vi "dosimat876_initialize.vi"(2 "error in":errorcluster, 3 "Dosimat Port In":refnum<visa-resource-name>="COM1") -> (1 "Dosimat Out":T1={"Dosimat Port out"="COM1", "Error out"={"status"=FALSE, "code"=0, "source"=""}})   [LabVIEW 2010]
uses:
  <vilib>/Instr/_visa.llb/VISA Configure Serial Port (Instr).vi
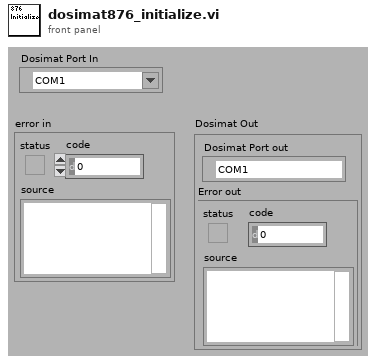
[diagram p1: front panel]
types:
  T1 = cluster{"Dosimat Port out":refnum<visa-resource-name>, "Error out":errorcluster}
  T2 = cluster{"Dosimat Port Out":refnum<visa-resource-name>, "error out":errorcluster}
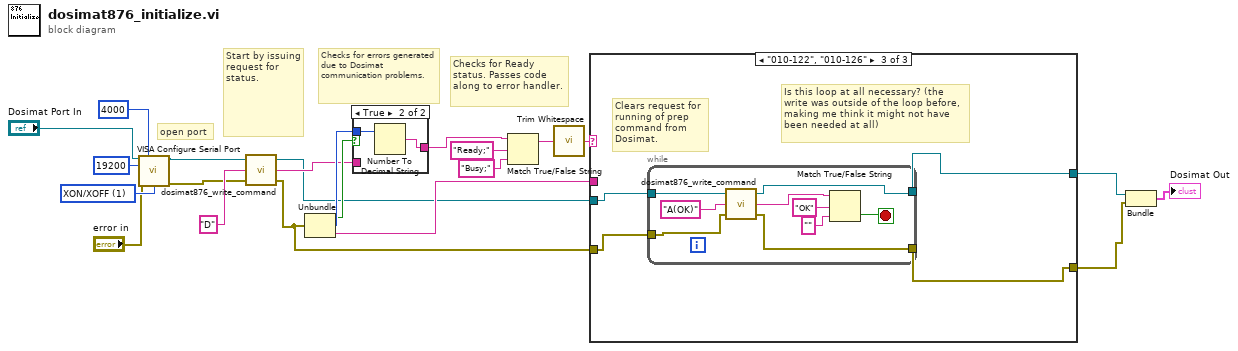
[diagram p0: block diagram]
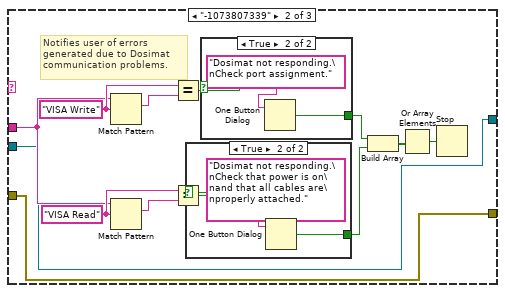
[diagram p4: hidden frame]
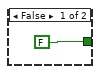
[diagram p5: hidden frame]
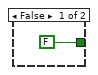
[diagram p6: hidden frame]
diagram:
  w6 = u16 1 items=["None", "XON/XOFF", "RTS/CTS", "XON/XOFF & RTS/CTS", "DTR/DSR", "XON/XOFF & DTR/DSR"] ("flow control (0:none)")
  # "open port"
  # "Checks for Ready status. Passes code along to error handler."
  # "Start by issuing request for status."
  # "Checks for errors generated due to Dosimat communication problems."
  n1 = call-poly "VISA Configure Serial Port"("VISA resource name"="Dosimat Port In", "timeout (10sec)"=u32 4000, "baud rate (9600)"=u32 19200, "error in (no error)"="error in", "flow control (0:none)"=w6) -> ("VISA resource name out"=w3:refnum<visa-resource-name>, "error out"=w2:errorcluster)  [unwired: 9 in]
  n2 = call "dosimat876_write_command.vi"("error in"=w2, "write buffer"="D", "Dosimat Port In"=w3) -> ("error out"=w11:errorcluster, "read buffer"=w18:string, "Dosimat Port Out"=w12:refnum<visa-resource-name>)
  n3 = Unbundle(w11) -> ("status"=w19:bool, "code"=w20:i32, "source"=w21:string)
  n4 = case shown="True" w19 {
    tunnel: w20 -> [_ w25]
    tunnel: [w23 w24] -> w14
    tunnel: w18 -> [w23 _]
    frame False {
    }
    frame True {
      n5 = Number To Decimal String(number=w25) -> (decimal integer string=w24:string)  [unwired: 1 in]
    }
  }
  n6 = Match True/False String(2:"Busy;" ("false string"), 3:"Ready;" ("true string"), 4:w14) -> (1:w15:string)  [unwired: 1 out]
  n7 = call <vilib>:"Trim Whitespace.vi"("string"=w15) -> ("trimmed string"=w13:string)  [unwired: 1 in]
  n8 = case shown="\"010-122\", \"010-126\"" w13 {
    tunnel: w21 -> [_ w34 _]
    tunnel: w12 -> [w27 w28 w50]
    tunnel: [w27 w28 w49] -> w9
    tunnel: [w26 w29 w47] -> w8
    tunnel: w11 -> [w26 w29 w48]
    frame "0", Default {
      # "No error detected yet."
    }
    frame "-1073807339" {
      w36 = "VISA Read" ("regular expression")
      w39 = "VISA Write" ("regular expression")
      # "Notifies user of errors generated due to Dosimat communication problems."
      n9 = Match Pattern(string=w34, regular expression=w39) -> (match substring=w40:string)  [unwired: 1 in, 3 out]
      n10 = Match Pattern(string=w34, regular expression=w36) -> (match substring=w35:string)  [unwired: 1 in, 3 out]
      n11 = Equal?(x=w39, y=w40) -> (x = y?=w38:bool)
      n12 = Equal?(x=w36, y=w35) -> (x = y?=w37:bool)
      n13 = case shown="True" w37 {
        tunnel: [FALSE w42] -> w32
        frame False {
        }
        frame True {
          n14 = One Button Dialog(message="Dosimat not responding.\nCheck that power is on\nand that all cables are\nproperly attached.") -> (true=w42:bool)  [unwired: 1 in]
        }
      }
      n15 = case shown="True" w38 {
        tunnel: [FALSE w45] -> w31
        frame False {
        }
        frame True {
          n16 = One Button Dialog(message="Dosimat not responding.\nCheck port assignment.") -> (true=w45:bool)  [unwired: 1 in]
        }
      }
      n17 = Build Array(w31, w32) -> (w30:bool[])
      n18 = Or Array Elements(Boolean array=w30) -> (logical OR=w33:bool)
      n19 = Stop(stop? (T)=w33) -> ()
    }
    frame "010-122", "010-126" {
      # "Is this loop at all necessary? (the write was outside of the loop before, making me think it might not have been needed at all)"
      # "Clears request for running of prep command from Dosimat."
      n20 = while {
        tunnel: w50 -> [w58]
        tunnel: [w57] -> w49
        tunnel: w48 -> [w56]
        tunnel: [w55] -> w47
        stop <- w51 stop-if-true
        n21 = call "dosimat876_write_command.vi"("error in"=w56, "write buffer"="A(OK)", "Dosimat Port In"=w58) -> ("error out"=w55:errorcluster, "read buffer"=w52:string, "Dosimat Port Out"=w57:refnum<visa-resource-name>)
        n22 = Match True/False String(2:"" ("false string"), 3:"OK" ("true string"), 4:w52) -> (0:w51:bool)  [unwired: 1 out]
      }
    }
  }
  n23 = Bundle("Dosimat Port Out"=w9, "error out"=w8) -> (→"Dosimat Out":T2)  [unwired: 1 in]
